vi "SP_OEE_2_test.vi"() -> ()   [LabVIEW 2017] (continued)
                      tunnel: [w12795] -> w12526
                      tunnel: [w12793] -> w12525
                      tunnel: [w12789] -> w12524
                      tunnel: [w12787] -> w12523
                      tunnel: w12538 -> [w12788]
                      tunnel: w12537 -> [w12784]
                      tunnel: [w12783] -> w12522
                      tunnel: w12536 -> [w12783]
                      tunnel: w12535 -> [w12844]
                      tunnel: w12534 -> [w12837]
                      tunnel: w12533 -> [w12828]
                      tunnel: w12532 -> [w12836]
                      tunnel: w12531 -> [w12826]
                      tunnel: w12530 -> [w12835]
                      tunnel: w12529 -> [w12824]
                      tunnel: w12528 -> [w12834]
                      tunnel: w12527 -> [w12822]
                      tunnel: w12526 -> [w12858]
                      tunnel: w12525 -> [w12857]
                      tunnel: w12524 -> [w12833]
                      tunnel: w12523 -> [w12820]
                      tunnel: [w12858] -> w12521
                      tunnel: [w12857] -> w12520
                      tunnel: [w12851] -> w12519
                      tunnel: [w12844] -> w12518
                      tunnel: [w12843] -> w12517
                      tunnel: [w12842] -> w12516
                      tunnel: [w12841] -> w12515
                      tunnel: [w12840] -> w12514
                      tunnel: [w12839] -> w12513
                      tunnel: [w12838] -> w12512
                      tunnel: [w12837] -> w12511
                      tunnel: [w12836] -> w12510
                      tunnel: [w12835] -> w12509
                      tunnel: [w12834] -> w12508
                      tunnel: [w12833] -> w12507
                      tunnel: [w12818] -> w12506
                      tunnel: w12522 -> [w12818]
                      tunnel: [w12859] -> _
                      tunnel: [w12868] -> w12497
                      tunnel: w12521 -> [w12869]
                      tunnel: w12520 -> [w12859]
                      tunnel: w12519 -> [w12863]
                      tunnel: w12518 -> [w12870]
                      tunnel: w12517 -> [_]
                      tunnel: w12516 -> [w12862]
                      tunnel: w12515 -> [_]
                      tunnel: w12514 -> [_]
                      tunnel: w12513 -> [_]
                      tunnel: w12512 -> [w12864]
                      tunnel: w12511 -> [_]
                      tunnel: w12510 -> [w12861]
                      tunnel: w12509 -> [_]
                      tunnel: w12508 -> [_]
                      tunnel: w12507 -> [_]
                      tunnel: w12506 -> [w12867]
                      tunnel: [w12859] -> w12496
                      frame #0 {
                        w12610 = "%Y-%m-%d" ("time format string (%c)")
                        n2295 = Decimal String To Number(string=w12596) -> (number=w12597:i32)  [unwired: 2 in, 1 out]
                        n2296 = property on="Table" class="Tbl (strict)"("Visible"=TRUE) -> ()  [unwired: 2 in, 2 out]
                        n2297 = Format Date/Time String(time format string (%c)=w12610, seconds (now)=w12602) -> (date/time string=w12611:string)  [unwired: 1 in]
                        n2298 = Format Date/Time String(time format string (%c)=w12610, seconds (now)=w12601) -> (date/time string=w12609:string)  [unwired: 1 in]
                        n2299 = Format Into String(format string="Where BREAKDOWN_DATE between '%s' and '%s' and  SHIFT_ID = '%d'  ", w12611, w12609, w12597) -> (resulting string=w12608:string)  [unwired: 2 in, 1 out]
                        n2300 = call <vilib>:"DB Tools Select Data.vi"("condition"=w12608, "error in (no error)"=w12617, "columns"=string[] ["BREAKDOWN_DATE"], "table"="STATION_1_LOG_HISTORY", "connection reference"=w12619) -> ("error out"=w12604:errorcluster, "data"=w12607:variant[][], "connection reference out"=w12618:T2)  [unwired: 1 in]
                        n2301 = property on="Table 2" class="Tbl (strict)"("Visible"=FALSE) -> ()  [unwired: 2 in, 2 out]
                        n2302 = xnode "Database Variant To Data"("database variant"=w12607, "error in (no error)"=w12604, "type"=string[][] [] ("Elements Found")) -> ("data"=w12605:string[][], "error out"=w12603:errorcluster)
                        n2303 = Index Array(array=w12605, index (col)=0 ("disabled index (col)")) -> (element=w12613:string[])  [unwired: 1 in]
                        n2304 = call "Search_1d_array_element.vi"("Count in"=string[] [] ("Elements Found"), "BD Date"=w12613, "Elements Found in"=string[] [] ("Elements Found")) -> ("Elements Found out"=w12600:string[])  [unwired: 4 in, 2 out]
                        n2305 = Build Array(w12600) -> (w12623:string[][])
                        n2306 = Transpose 2D Array(2D array=w12623) -> (transposed array=w12622:string[][])
                      }
                      frame #1 {
                        n2307 = disable-structure shown="Enabled" {
                          disable-tunnel: w12685 -> [w12696 w12698]
                          disable-tunnel: [w12695 w12698] -> w12684
                          disable-tunnel: w12683 -> [w12694 w12699]
                          disable-tunnel: [w12693 w12699] -> w12682
                          disable-tunnel: w12680 -> [w12691 _]
                          disable-tunnel: w12679 -> [w12690 _]
                          disable-tunnel: [w12689 _] -> w12678
                          disable-tunnel: [w12688 _] -> w12675
                          disable-tunnel: w12673 -> [w12687 _]
                          disable-tunnel: w12670 -> [w12686 w12697]
                          disable-tunnel: [_ w12697] -> w12669
                          frame Disabled {
                            n2308 = call "Stack_holderwise_total_bd_count_&_duration_2.vi"("Refnum in"=w12696, "BREAKDOWN_STK_HOLD_ID"=1, "condition"=w12687, "Form Date"=w12691, "To Date"=w12690, "error in (no error)"=w12694, "Shift"=w12686) -> ("Refnum out"=w12695:T2, "Count out"=w12689:string[], "appended array"=w12688:dbl[], "error out"=w12693:errorcluster)  [unwired: 5 in]
                          }
                          frame Enabled {
                          }
                        }
                        n2309 = call "NUMERIC TO STRING.vi"("appended array"=w12675) -> ("Array"=w12674:string[])  [unwired: 4 in]
                        n2310 = call "Insert_empty_element_with_zero.vi"("searched date"=w12678, "fixed date"=w12676) -> ("O/P"=w12671:string[])  [unwired: 9 in]
                        n2311 = call "Insert_empty_element_with_zero.vi"("searched date"=w12674, "fixed date"=w12676) -> ("O/P"=w12677:string[])  [unwired: 9 in]
                      }
                      frame #2 {
                        n2312 = call "Stack_holderwise_total_bd_count_&_duration_2.vi"("Refnum in"=w12713, "BREAKDOWN_STK_HOLD_ID"=2, "condition"=w12703, "Form Date"=w12711, "To Date"=w12710, "error in (no error)"=w12715, "Shift"=w12700) -> ("Refnum out"=w12712:T2, "Count out"=w12709:string[], "appended array"=w12705:dbl[], "error out"=w12714:errorcluster)  [unwired: 5 in]
                        n2313 = call "Insert_empty_element_with_zero.vi"("searched date"=w12709, "fixed date"=w12706) -> ("O/P"=w12708:string[])  [unwired: 9 in]
                        n2314 = call "NUMERIC TO STRING.vi"("appended array"=w12705) -> ("Array"=w12704:string[])  [unwired: 4 in]
                        n2315 = call "Insert_empty_element_with_zero.vi"("searched date"=w12704, "fixed date"=w12706) -> ("O/P"=w12707:string[])  [unwired: 9 in]
                      }
                      frame #3 {
                        n2316 = disable-structure shown="Enabled" {
                          disable-tunnel: w12732 -> [w12746 w12749]
                          disable-tunnel: [w12745 w12749] -> w12731
                          disable-tunnel: w12730 -> [w12744 w12748]
                          disable-tunnel: [w12743 w12748] -> w12729
                          disable-tunnel: w12728 -> [w12742 _]
                          disable-tunnel: w12727 -> [w12741 _]
                          disable-tunnel: [w12740 _] -> w12726
                          disable-tunnel: [w12739 _] -> w12722
                          disable-tunnel: w12720 -> [w12738 _]
                          frame Disabled {
                            n2317 = call "Stack_holderwise_total_bd_count_&_duration.vi"("Refnum in"=w12744, "BREAKDOWN_STK_HOLD_ID"=3, "condition"=w12738, "Form Date"=w12742, "To Date"=w12741, "error in (no error)"=w12746) -> ("Refnum out"=w12743:T2, "Count out"=w12740:string[], "appended array"=w12739:dbl[], "error out"=w12745:errorcluster)  [unwired: 6 in]
                          }
                          frame Enabled {
                          }
                        }
                        n2318 = call "Insert_empty_element_with_zero.vi"("searched date"=w12726, "fixed date"=w12723) -> ("O/P"=w12725:string[])  [unwired: 9 in]
                        n2319 = call "NUMERIC TO STRING.vi"("appended array"=w12722) -> ("Array"=w12721:string[])  [unwired: 4 in]
                        n2320 = call "Insert_empty_element_with_zero.vi"("searched date"=w12721, "fixed date"=w12723) -> ("O/P"=w12724:string[])  [unwired: 9 in]
                      }
                      frame #4 {
                        n2321 = disable-structure shown="Enabled" {
                          disable-tunnel: w12763 -> [w12779 w12782]
                          disable-tunnel: w12762 -> [w12778 w12781]
                          disable-tunnel: [w12777 w12781] -> w12761
                          disable-tunnel: [w12776 w12782] -> w12760
                          disable-tunnel: w12759 -> [w12775 _]
                          disable-tunnel: w12758 -> [w12774 _]
                          disable-tunnel: [w12773 _] -> w12757
                          disable-tunnel: [w12772 _] -> w12753
                          disable-tunnel: w12751 -> [w12771 _]
                          frame Disabled {
                            n2322 = call "Stack_holderwise_total_bd_count_&_duration.vi"("Refnum in"=w12778, "BREAKDOWN_STK_HOLD_ID"=4, "condition"=w12771, "Form Date"=w12775, "To Date"=w12774, "error in (no error)"=w12779) -> ("Refnum out"=w12777:T2, "Count out"=w12773:string[], "appended array"=w12772:dbl[], "error out"=w12776:errorcluster)  [unwired: 6 in]
                          }
                          frame Enabled {
                          }
                        }
                        n2323 = call "Insert_empty_element_with_zero.vi"("searched date"=w12757, "fixed date"=w12754) -> ("O/P"=w12756:string[])  [unwired: 9 in]
                        n2324 = call "NUMERIC TO STRING.vi"("appended array"=w12753) -> ("Array"=w12752:string[])  [unwired: 4 in]
                        n2325 = call "Insert_empty_element_with_zero.vi"("searched date"=w12752, "fixed date"=w12754) -> ("O/P"=w12755:string[])  [unwired: 9 in]
                      }
                      frame #5 {
                        n2326 = disable-structure shown="Enabled" {
                          disable-tunnel: w12796 -> [w12814 w12817]
                          disable-tunnel: [w12813 w12817] -> w12795
                          disable-tunnel: w12794 -> [w12812 w12816]
                          disable-tunnel: [w12811 w12816] -> w12793
                          disable-tunnel: w12792 -> [w12810 _]
                          disable-tunnel: w12791 -> [w12809 _]
                          disable-tunnel: [w12808 _] -> w12790
                          disable-tunnel: [w12807 _] -> w12786
                          disable-tunnel: w12784 -> [w12806 _]
                          frame Disabled {
                            n2327 = call "Stack_holderwise_total_bd_count_&_duration.vi"("Refnum in"=w12812, "BREAKDOWN_STK_HOLD_ID"=5, "condition"=w12806, "Form Date"=w12809, "To Date"=w12810, "error in (no error)"=w12814) -> ("Refnum out"=w12811:T2, "Count out"=w12808:string[], "appended array"=w12807:dbl[], "error out"=w12813:errorcluster)  [unwired: 6 in]
                          }
                          frame Enabled {
                          }
                        }
                        n2328 = call "NUMERIC TO STRING.vi"("appended array"=w12786) -> ("Array"=w12785:string[])  [unwired: 4 in]
                        n2329 = call "Insert_empty_element_with_zero.vi"("searched date"=w12790, "fixed date"=w12788) -> ("O/P"=w12789:string[])  [unwired: 9 in]
                        n2330 = call "Insert_empty_element_with_zero.vi"("searched date"=w12785, "fixed date"=w12788) -> ("O/P"=w12787:string[])  [unwired: 9 in]
                      }
                      frame #6 {
                        n2331 = call "String to numeric.vi"("Array"=w12828) -> ("Array 2"=w12827:dbl[])  [unwired: 4 in]
                        n2332 = call "String to numeric.vi"("Array"=w12826) -> ("Array 2"=w12825:dbl[])  [unwired: 4 in]
                        n2333 = call "String to numeric.vi"("Array"=w12824) -> ("Array 2"=w12823:dbl[])  [unwired: 4 in]
                        n2334 = call "String to numeric.vi"("Array"=w12822) -> ("Array 2"=w12821:dbl[])  [unwired: 4 in]
                        n2335 = call "String to numeric.vi"("Array"=w12820) -> ("Array 2"=w12819:dbl[])  [unwired: 4 in]
                        n2336 = Decimal String To Number(string=w12833) -> (number=w12852:i32[])  [unwired: 2 in, 1 out]
                        n2337 = Decimal String To Number(string=w12834) -> (number=w12853:i32[])  [unwired: 2 in, 1 out]
                        n2338 = Decimal String To Number(string=w12835) -> (number=w12854:i32[])  [unwired: 2 in, 1 out]
                        n2339 = Decimal String To Number(string=w12836) -> (number=w12855:i32[])  [unwired: 2 in, 1 out]
                        n2340 = Decimal String To Number(string=w12837) -> (number=w12850:i32[])  [unwired: 2 in, 1 out]
                        n2341 = Compound Arithmetic op=ADD(w12827, w12825, w12823, w12821, w12819) -> (w12830:dbl[])
                        n2342 = Build Array(w12828) -> (w12849:string[][])
                        n2343 = Build Array(w12826) -> (w12848:string[][])
                        n2344 = Build Array(w12824) -> (w12847:string[][])
                        n2345 = Build Array(w12822) -> (w12846:string[][])
                        n2346 = Build Array(w12820) -> (w12845:string[][])
                        n2347 = Number To Fractional String(number=w12830, precision (6)=i16 2) -> (F-format string=w12829:string[])  [unwired: 2 in]
                        n2348 = Compound Arithmetic op=ADD(w12852, w12853, w12854, w12855, w12850) -> (w12856:i32[])
                        n2349 = Transpose 2D Array(2D array=w12849) -> (transposed array=w12843:string[][])
                        n2350 = Transpose 2D Array(2D array=w12848) -> (transposed array=w12842:string[][])
                        n2351 = Transpose 2D Array(2D array=w12847) -> (transposed array=w12841:string[][])
                        n2352 = Transpose 2D Array(2D array=w12846) -> (transposed array=w12840:string[][])
                        n2353 = Transpose 2D Array(2D array=w12845) -> (transposed array=w12839:string[][])
                        n2354 = Number To Decimal String(number=w12856) -> (decimal integer string=w12851:string[])  [unwired: 1 in]
                        n2355 = Build Array(w12829) -> (w12832:string[][])
                        n2356 = Transpose 2D Array(2D array=w12832) -> (transposed array=w12838:string[][])
                      }
                      frame #7 {
                        w12860 = string[] [""]
                        n2357 = Insert Into Array(array=w12870, index (col)=1 ("disabled index (col)"), new element #1=w12860, new element #2=w12860, new element #3=w12861, new element #4=w12862, new element #5=w12860, new element #6=w12860, new element #7=w12860, new element #8=w12860, new element #9=w12860, new element #10=w12860, new element #11=w12863, new element #12=w12864) -> (w12866:string[][])  [unwired: 1 in]
                        n2358 = call "flot graph for month n year.vi"("BD Date"=w12867, "error in (no error)"=w12869, "Count total"=w12863) -> ("error out"=w12868:errorcluster, "Run-Time Status"=w12865:cluster{"Array 2":timestamp[], dbl[]})  [unwired: 7 in]
                        n2359 = local write "Run-Time Status"(w12865) -> ()
                        n2360 = local write "Table"(w12866) -> ()
                      }
                    }
                  }
                  frame "2" {
                    n2361 = flat-sequence {
                      tunnel: w12879 -> [w12993]
                      tunnel: w12878 -> [w12991]
                      tunnel: [w12977] -> w12969
                      tunnel: [w12992] -> w12968
                      tunnel: w12877 -> [_]
                      tunnel: [w12996] -> w12967
                      tunnel: [w12976] -> w12966
                      tunnel: [w12975] -> w12965
                      tunnel: [w12974] -> w12964
                      tunnel: w12876 -> [w12976]
                      tunnel: w12875 -> [w12975]
                      tunnel: ["Where BREAKDOWN_DATE between '%s'and '%s' and BREAKDOWN_STK_HOLD_ID ='%d' and  SHIFT_ID = '%d' "] -> w12963
                      tunnel: [w12974] -> w12962
                      tunnel: w12874 -> [w12970]
                      tunnel: [w12970] -> w12873
                      tunnel: w12969 -> [w13057]
                      tunnel: w12968 -> [w13059]
                      tunnel: w12967 -> [w13055]
                      tunnel: w12966 -> [w13054]
                      tunnel: w12965 -> [w13053]
                      tunnel: [w13056] -> w12961
                      tunnel: [w13058] -> w12960
                      tunnel: [w13055] -> w12959
                      tunnel: [w13045] -> w12958
                      tunnel: [w13051] -> w12957
                      tunnel: [w13054] -> w12956
                      tunnel: [w13053] -> w12955
                      tunnel: w12964 -> [w13050]
                      tunnel: [w13050] -> w12954
                      tunnel: w12963 -> [w13047]
                      tunnel: [w13047] -> w12953
                      tunnel: [w13046] -> w12952
                      tunnel: w12962 -> [w13046]
                      tunnel: w12873 -> [w13044]
                      tunnel: [w13043] -> w12872
                      tunnel: w12961 -> [w13089]
                      tunnel: w12960 -> [w13087]
                      tunnel: w12959 -> [w13092]
                      tunnel: w12958 -> [w13091]
                      tunnel: w12957 -> [w13090]
                      tunnel: w12956 -> [w13085]
                      tunnel: w12955 -> [w13084]
                      tunnel: [w13092] -> w12951
                      tunnel: [w13091] -> w12950
                      tunnel: [w13090] -> w12949
                      tunnel: [w13088] -> w12948
                      tunnel: [w13082] -> w12947
                      tunnel: [w13081] -> w12946
                      tunnel: [w13086] -> w12945
                      tunnel: [w13085] -> w12944
                      tunnel: [w13084] -> w12943
                      tunnel: w12954 -> [w13080]
                      tunnel: [w13080] -> w12942
                      tunnel: w12953 -> [w13077]
                      tunnel: [w13077] -> w12941
                      tunnel: [w13076] -> w12940
                      tunnel: w12952 -> [w13076]
                      tunnel: w12872 -> [w13074]
                      tunnel: w12951 -> [w13111]
                      tunnel: w12950 -> [w13110]
                      tunnel: w12949 -> [w13109]
                      tunnel: w12948 -> [w13106]
                      tunnel: w12947 -> [w13108]
                      tunnel: w12946 -> [w13107]
                      tunnel: w12945 -> [w13104]
                      tunnel: w12944 -> [w13102]
                      tunnel: w12943 -> [w13101]
                      tunnel: [w13111] -> w12939
                      tunnel: [w13110] -> w12938
                      tunnel: [w13109] -> w12937
                      tunnel: [w13108] -> w12936
                      tunnel: [w13107] -> w12935
                      tunnel: [w13105] -> w12934
                      tunnel: [w13099] -> w12933
                      tunnel: [w13098] -> w12932
                      tunnel: [w13103] -> w12931
                      tunnel: [w13102] -> w12930
                      tunnel: [w13101] -> w12929
                      tunnel: w12942 -> [w13097]
                      tunnel: [w13097] -> w12928
                      tunnel: w12941 -> [w13094]
                      tunnel: [w13094] -> w12927
                      tunnel: [w13093] -> w12926
                      tunnel: w12940 -> [w13093]
                      tunnel: w12939 -> [w13144]
                      tunnel: w12938 -> [w13143]
                      tunnel: w12937 -> [w13142]
                      tunnel: w12936 -> [w13141]
                      tunnel: w12935 -> [w13140]
                      tunnel: w12934 -> [w13137]
                      tunnel: w12933 -> [w13139]
                      tunnel: w12932 -> [w13138]
                      tunnel: w12931 -> [w13136]
                      tunnel: w12930 -> [w13133]
                      tunnel: w12929 -> [w13132]
                      tunnel: [w13144] -> w12925
                      tunnel: [w13143] -> w12924
                      tunnel: [w13142] -> w12923
                      tunnel: [w13141] -> w12922
                      tunnel: [w13140] -> w12921
                      tunnel: [w13139] -> w12920
                      tunnel: [w13138] -> w12919
                      tunnel: [w13135] -> w12918
                      tunnel: [w13134] -> w12917
                      tunnel: [w13130] -> w12916
                      tunnel: [w13129] -> w12915
                      tunnel: [w13133] -> w12914
                      tunnel: [w13132] -> w12913
                      tunnel: w12928 -> [w13128]
                      tunnel: [w13128] -> w12912
                      tunnel: w12927 -> [w13125]
                      tunnel: [w13125] -> w12911
                      tunnel: [w13124] -> w12910
                      tunnel: w12926 -> [w13124]
                      tunnel: w12925 -> [w13179]
                      tunnel: w12924 -> [w13178]
                      tunnel: w12923 -> [w13177]
                      tunnel: w12922 -> [w13176]
                      tunnel: w12921 -> [w13175]
                      tunnel: w12920 -> [w13174]
                      tunnel: w12919 -> [w13173]
                      tunnel: w12918 -> [w13168]
                      tunnel: w12917 -> [w13170]
                      tunnel: w12916 -> [w13172]
                      tunnel: w12915 -> [w13171]
                      tunnel: w12914 -> [w13165]
                      tunnel: w12913 -> [w13166]
                      tunnel: [w13179] -> w12909
                      tunnel: [w13178] -> w12908
                      tunnel: [w13177] -> w12907
                      tunnel: [w13176] -> w12906
                      tunnel: [w13175] -> w12905
                      tunnel: [w13174] -> w12904
                      tunnel: [w13173] -> w12903
                      tunnel: [w13172] -> w12902
                      tunnel: [w13171] -> w12901
                      tunnel: [w13169] -> w12900
                      tunnel: [w13167] -> w12899
                      tunnel: [w13163] -> w12898
                      tunnel: [w13161] -> w12897
                      tunnel: w12912 -> [w13162]
                      tunnel: w12911 -> [w13158]
                      tunnel: [w13157] -> w12896
                      tunnel: w12910 -> [w13157]
                      tunnel: w12909 -> [w13218]
                      tunnel: w12908 -> [w13211]
                      tunnel: w12907 -> [w13202]
                      tunnel: w12906 -> [w13210]
                      tunnel: w12905 -> [w13200]
                      tunnel: w12904 -> [w13209]
                      tunnel: w12903 -> [w13198]
                      tunnel: w12902 -> [w13208]
                      tunnel: w12901 -> [w13196]
                      tunnel: w12900 -> [w13232]
                      tunnel: w12899 -> [w13231]
                      tunnel: w12898 -> [w13207]
                      tunnel: w12897 -> [w13194]
                      tunnel: [w13232] -> w12895
                      tunnel: [w13231] -> w12894
                      tunnel: [w13225] -> w12893
                      tunnel: [w13218] -> w12892
                      tunnel: [w13217] -> w12891
                      tunnel: [w13216] -> w12890
                      tunnel: [w13215] -> w12889
                      tunnel: [w13214] -> w12888
                      tunnel: [w13213] -> w12887
                      tunnel: [w13212] -> w12886
                      tunnel: [w13211] -> w12885
                      tunnel: [w13210] -> w12884
                      tunnel: [w13209] -> w12883
                      tunnel: [w13208] -> w12882
                      tunnel: [w13207] -> w12881
                      tunnel: [w13192] -> w12880
                      tunnel: w12896 -> [w13192]
                      tunnel: [w13245] -> _
                      tunnel: [w13241] -> _
                      tunnel: w12895 -> [w13242]
                      tunnel: w12894 -> [w13245]
                      tunnel: w12893 -> [w13236]
                      tunnel: w12892 -> [w13243]
                      tunnel: w12891 -> [_]
                      tunnel: w12890 -> [w13235]
                      tunnel: w12889 -> [_]
                      tunnel: w12888 -> [_]
                      tunnel: w12887 -> [_]
                      tunnel: w12886 -> [w13237]
                      tunnel: w12885 -> [_]
                      tunnel: w12884 -> [w13234]
                      tunnel: w12883 -> [_]
                      tunnel: w12882 -> [_]
                      tunnel: w12881 -> [_]
                      tunnel: w12880 -> [w13240]
                      frame #0 {
                        w12984 = "%Y-%m-%d" ("time format string (%c)")
                        n2362 = Decimal String To Number(string=w12970) -> (number=w12971:i32)  [unwired: 2 in, 1 out]
                        n2363 = property on="Table" class="Tbl (strict)"("Visible"=TRUE) -> ()  [unwired: 2 in, 2 out]
                        n2364 = Format Date/Time String(time format string (%c)=w12984, seconds (now)=w12976) -> (date/time string=w12985:string)  [unwired: 1 in]
                        n2365 = Format Date/Time String(time format string (%c)=w12984, seconds (now)=w12975) -> (date/time string=w12983:string)  [unwired: 1 in]
                        n2366 = Format Into String(format string="Where BREAKDOWN_DATE between '%s' and '%s' and  SHIFT_ID = '%d'  ", w12985, w12983, w12971) -> (resulting string=w12982:string)  [unwired: 2 in, 1 out]
                        n2367 = call <vilib>:"DB Tools Select Data.vi"("condition"=w12982, "error in (no error)"=w12991, "columns"=string[] ["BREAKDOWN_DATE"], "table"="STATION_1_LOG_HISTORY", "connection reference"=w12993) -> ("error out"=w12978:errorcluster, "data"=w12981:variant[][], "connection reference out"=w12992:T2)  [unwired: 1 in]
                        n2368 = property on="Table 2" class="Tbl (strict)"("Visible"=FALSE) -> ()  [unwired: 2 in, 2 out]
                        n2369 = xnode "Database Variant To Data"("database variant"=w12981, "error in (no error)"=w12978, "type"=string[][] [] ("Elements Found")) -> ("data"=w12979:string[][], "error out"=w12977:errorcluster)
                        n2370 = Index Array(array=w12979, index (col)=0 ("disabled index (col)")) -> (element=w12987:string[])  [unwired: 1 in]
                        n2371 = call "Search_1d_array_element.vi"("Count in"=string[] [] ("Elements Found"), "BD Date"=w12987, "Elements Found in"=string[] [] ("Elements Found")) -> ("Elements Found out"=w12974:string[])  [unwired: 4 in, 2 out]
                        n2372 = Build Array(w12974) -> (w12997:string[][])
                        n2373 = Transpose 2D Array(2D array=w12997) -> (transposed array=w12996:string[][])
                      }
                      frame #1 {
                        n2374 = disable-structure shown="Enabled" {
                          disable-tunnel: w13059 -> [w13070 w13072]
                          disable-tunnel: [w13069 w13072] -> w13058
                          disable-tunnel: w13057 -> [w13068 w13073]
                          disable-tunnel: [w13067 w13073] -> w13056
                          disable-tunnel: w13054 -> [w13065 _]
                          disable-tunnel: w13053 -> [w13064 _]
                          disable-tunnel: [w13063 _] -> w13052
                          disable-tunnel: [w13062 _] -> w13049
                          disable-tunnel: w13047 -> [w13061 _]
                          disable-tunnel: w13044 -> [w13060 w13071]
                          disable-tunnel: [_ w13071] -> w13043
                          frame Disabled {
                            n2375 = call "Stack_holderwise_total_bd_count_&_duration_2.vi"("Refnum in"=w13070, "BREAKDOWN_STK_HOLD_ID"=1, "condition"=w13061, "Form Date"=w13065, "To Date"=w13064, "error in (no error)"=w13068, "Shift"=w13060) -> ("Refnum out"=w13069:T2, "Count out"=w13063:string[], "appended array"=w13062:dbl[], "error out"=w13067:errorcluster)  [unwired: 5 in]
                          }
                          frame Enabled {
                          }
                        }
                        n2376 = call "NUMERIC TO STRING.vi"("appended array"=w13049) -> ("Array"=w13048:string[])  [unwired: 4 in]
                        n2377 = call "Insert_empty_element_with_zero.vi"("searched date"=w13052, "fixed date"=w13050) -> ("O/P"=w13045:string[])  [unwired: 9 in]
                        n2378 = call "Insert_empty_element_with_zero.vi"("searched date"=w13048, "fixed date"=w13050) -> ("O/P"=w13051:string[])  [unwired: 9 in]
                      }
                      frame #2 {
                        n2379 = call "Stack_holderwise_total_bd_count_&_duration_2.vi"("Refnum in"=w13087, "BREAKDOWN_STK_HOLD_ID"=2, "condition"=w13077, "Form Date"=w13085, "To Date"=w13084, "error in (no error)"=w13089, "Shift"=w13074) -> ("Refnum out"=w13086:T2, "Count out"=w13083:string[], "appended array"=w13079:dbl[], "error out"=w13088:errorcluster)  [unwired: 5 in]
                        n2380 = call "Insert_empty_element_with_zero.vi"("searched date"=w13083, "fixed date"=w13080) -> ("O/P"=w13082:string[])  [unwired: 9 in]
                        n2381 = call "NUMERIC TO STRING.vi"("appended array"=w13079) -> ("Array"=w13078:string[])  [unwired: 4 in]
                        n2382 = call "Insert_empty_element_with_zero.vi"("searched date"=w13078, "fixed date"=w13080) -> ("O/P"=w13081:string[])  [unwired: 9 in]
                      }
                      frame #3 {
                        n2383 = disable-structure shown="Enabled" {
                          disable-tunnel: w13106 -> [w13120 w13123]
                          disable-tunnel: [w13119 w13123] -> w13105
                          disable-tunnel: w13104 -> [w13118 w13122]
                          disable-tunnel: [w13117 w13122] -> w13103
                          disable-tunnel: w13102 -> [w13116 _]
                          disable-tunnel: w13101 -> [w13115 _]
                          disable-tunnel: [w13114 _] -> w13100
                          disable-tunnel: [w13113 _] -> w13096
                          disable-tunnel: w13094 -> [w13112 _]
                          frame Disabled {
                            n2384 = call "Stack_holderwise_total_bd_count_&_duration.vi"("Refnum in"=w13118, "BREAKDOWN_STK_HOLD_ID"=3, "condition"=w13112, "Form Date"=w13116, "To Date"=w13115, "error in (no error)"=w13120) -> ("Refnum out"=w13117:T2, "Count out"=w13114:string[], "appended array"=w13113:dbl[], "error out"=w13119:errorcluster)  [unwired: 6 in]
                          }
                          frame Enabled {
                          }
                        }
                        n2385 = call "Insert_empty_element_with_zero.vi"("searched date"=w13100, "fixed date"=w13097) -> ("O/P"=w13099:string[])  [unwired: 9 in]
                        n2386 = call "NUMERIC TO STRING.vi"("appended array"=w13096) -> ("Array"=w13095:string[])  [unwired: 4 in]
                        n2387 = call "Insert_empty_element_with_zero.vi"("searched date"=w13095, "fixed date"=w13097) -> ("O/P"=w13098:string[])  [unwired: 9 in]
                      }
                      frame #4 {
                        n2388 = disable-structure shown="Enabled" {
                          disable-tunnel: w13137 -> [w13153 w13156]
                          disable-tunnel: w13136 -> [w13152 w13155]
                          disable-tunnel: [w13151 w13155] -> w13135
                          disable-tunnel: [w13150 w13156] -> w13134
                          disable-tunnel: w13133 -> [w13149 _]
                          disable-tunnel: w13132 -> [w13148 _]
                          disable-tunnel: [w13147 _] -> w13131
                          disable-tunnel: [w13146 _] -> w13127
                          disable-tunnel: w13125 -> [w13145 _]
                          frame Disabled {
                            n2389 = call "Stack_holderwise_total_bd_count_&_duration.vi"("Refnum in"=w13152, "BREAKDOWN_STK_HOLD_ID"=4, "condition"=w13145, "Form Date"=w13149, "To Date"=w13148, "error in (no error)"=w13153) -> ("Refnum out"=w13151:T2, "Count out"=w13147:string[], "appended array"=w13146:dbl[], "error out"=w13150:errorcluster)  [unwired: 6 in]
                          }
                          frame Enabled {
                          }
                        }
                        n2390 = call "Insert_empty_element_with_zero.vi"("searched date"=w13131, "fixed date"=w13128) -> ("O/P"=w13130:string[])  [unwired: 9 in]
                        n2391 = call "NUMERIC TO STRING.vi"("appended array"=w13127) -> ("Array"=w13126:string[])  [unwired: 4 in]
                        n2392 = call "Insert_empty_element_with_zero.vi"("searched date"=w13126, "fixed date"=w13128) -> ("O/P"=w13129:string[])  [unwired: 9 in]
                      }
                      frame #5 {
                        n2393 = disable-structure shown="Enabled" {
                          disable-tunnel: w13170 -> [w13188 w13191]
                          disable-tunnel: [w13187 w13191] -> w13169
                          disable-tunnel: w13168 -> [w13186 w13190]
                          disable-tunnel: [w13185 w13190] -> w13167
                          disable-tunnel: w13166 -> [w13184 _]
                          disable-tunnel: w13165 -> [w13183 _]
                          disable-tunnel: [w13182 _] -> w13164
                          disable-tunnel: [w13181 _] -> w13160
                          disable-tunnel: w13158 -> [w13180 _]
                          frame Disabled {
                            n2394 = call "Stack_holderwise_total_bd_count_&_duration.vi"("Refnum in"=w13186, "BREAKDOWN_STK_HOLD_ID"=5, "condition"=w13180, "Form Date"=w13183, "To Date"=w13184, "error in (no error)"=w13188) -> ("Refnum out"=w13185:T2, "Count out"=w13182:string[], "appended array"=w13181:dbl[], "error out"=w13187:errorcluster)  [unwired: 6 in]
                          }
                          frame Enabled {
                          }
                        }
                        n2395 = call "NUMERIC TO STRING.vi"("appended array"=w13160) -> ("Array"=w13159:string[])  [unwired: 4 in]
                        n2396 = call "Insert_empty_element_with_zero.vi"("searched date"=w13164, "fixed date"=w13162) -> ("O/P"=w13163:string[])  [unwired: 9 in]
                        n2397 = call "Insert_empty_element_with_zero.vi"("searched date"=w13159, "fixed date"=w13162) -> ("O/P"=w13161:string[])  [unwired: 9 in]
                      }
                      frame #6 {
                        n2398 = call "String to numeric.vi"("Array"=w13202) -> ("Array 2"=w13201:dbl[])  [unwired: 4 in]
                        n2399 = call "String to numeric.vi"("Array"=w13200) -> ("Array 2"=w13199:dbl[])  [unwired: 4 in]
                        n2400 = call "String to numeric.vi"("Array"=w13198) -> ("Array 2"=w13197:dbl[])  [unwired: 4 in]
                        n2401 = call "String to numeric.vi"("Array"=w13196) -> ("Array 2"=w13195:dbl[])  [unwired: 4 in]
                        n2402 = call "String to numeric.vi"("Array"=w13194) -> ("Array 2"=w13193:dbl[])  [unwired: 4 in]
                        n2403 = Decimal String To Number(string=w13207) -> (number=w13226:i32[])  [unwired: 2 in, 1 out]
                        n2404 = Decimal String To Number(string=w13208) -> (number=w13227:i32[])  [unwired: 2 in, 1 out]
                        n2405 = Decimal String To Number(string=w13209) -> (number=w13228:i32[])  [unwired: 2 in, 1 out]
                        n2406 = Decimal String To Number(string=w13210) -> (number=w13229:i32[])  [unwired: 2 in, 1 out]
                        n2407 = Decimal String To Number(string=w13211) -> (number=w13224:i32[])  [unwired: 2 in, 1 out]
                        n2408 = Compound Arithmetic op=ADD(w13201, w13199, w13197, w13195, w13193) -> (w13204:dbl[])
                        n2409 = Build Array(w13202) -> (w13223:string[][])
                        n2410 = Build Array(w13200) -> (w13222:string[][])
                        n2411 = Build Array(w13198) -> (w13221:string[][])
                        n2412 = Build Array(w13196) -> (w13220:string[][])
                        n2413 = Build Array(w13194) -> (w13219:string[][])
                        n2414 = Number To Fractional String(number=w13204, precision (6)=i16 2) -> (F-format string=w13203:string[])  [unwired: 2 in]
                        n2415 = Compound Arithmetic op=ADD(w13226, w13227, w13228, w13229, w13224) -> (w13230:i32[])
                        n2416 = Transpose 2D Array(2D array=w13223) -> (transposed array=w13217:string[][])
                        n2417 = Transpose 2D Array(2D array=w13222) -> (transposed array=w13216:string[][])
                        n2418 = Transpose 2D Array(2D array=w13221) -> (transposed array=w13215:string[][])
                        n2419 = Transpose 2D Array(2D array=w13220) -> (transposed array=w13214:string[][])
                        n2420 = Transpose 2D Array(2D array=w13219) -> (transposed array=w13213:string[][])
                        n2421 = Number To Decimal String(number=w13230) -> (decimal integer string=w13225:string[])  [unwired: 1 in]
                        n2422 = Build Array(w13203) -> (w13206:string[][])
                        n2423 = Transpose 2D Array(2D array=w13206) -> (transposed array=w13212:string[][])
                      }
                      frame #7 {
                        w13233 = string[] [""]
                        n2424 = Insert Into Array(array=w13243, index (col)=1 ("disabled index (col)"), new element #1=w13233, new element #2=w13233, new element #3=w13234, new element #4=w13235, new element #5=w13233, new element #6=w13233, new element #7=w13233, new element #8=w13233, new element #9=w13233, new element #10=w13233, new element #11=w13236, new element #12=w13237) -> (w13239:string[][])  [unwired: 1 in]
                        n2425 = call "flot graph for month n year.vi"("BD Date"=w13240, "error in (no error)"=w13242, "Count total"=w13236) -> ("error out"=w13241:errorcluster, "Run-Time Status"=w13238:cluster{"Array 2":timestamp[], dbl[]})  [unwired: 7 in]
                        n2426 = local write "Run-Time Status"(w13238) -> ()
                        n2427 = local write "Table"(w13239) -> ()
                      }
                    }
                  }
                  frame "3" {
                    n2428 = flat-sequence {
                      tunnel: w13253 -> [w13367]
                      tunnel: w13252 -> [w13365]
                      tunnel: [w13351] -> w13343
                      tunnel: [w13366] -> w13342
                      tunnel: w13251 -> [_]
                      tunnel: [w13370] -> w13341
                      tunnel: [w13350] -> w13340
                      tunnel: [w13349] -> w13339
                      tunnel: [w13348] -> w13338
                      tunnel: w13250 -> [w13350]
                      tunnel: w13249 -> [w13349]
                      tunnel: ["Where BREAKDOWN_DATE between '%s'and '%s' and BREAKDOWN_STK_HOLD_ID ='%d' and  SHIFT_ID = '%d' "] -> w13337
                      tunnel: [w13348] -> w13336
                      tunnel: w13248 -> [w13344]
                      tunnel: [w13344] -> w13247
                      tunnel: w13343 -> [w13431]
                      tunnel: w13342 -> [w13433]
                      tunnel: w13341 -> [w13429]
                      tunnel: w13340 -> [w13428]
                      tunnel: w13339 -> [w13427]
                      tunnel: [w13430] -> w13335
                      tunnel: [w13432] -> w13334
                      tunnel: [w13429] -> w13333
                      tunnel: [w13419] -> w13332
                      tunnel: [w13425] -> w13331
                      tunnel: [w13428] -> w13330
                      tunnel: [w13427] -> w13329
                      tunnel: w13338 -> [w13424]
                      tunnel: [w13424] -> w13328
                      tunnel: w13337 -> [w13421]
                      tunnel: [w13421] -> w13327
                      tunnel: [w13420] -> w13326
                      tunnel: w13336 -> [w13420]
                      tunnel: w13247 -> [w13418]
                      tunnel: [w13417] -> w13246
                      tunnel: w13335 -> [w13463]
                      tunnel: w13334 -> [w13461]
                      tunnel: w13333 -> [w13466]
                      tunnel: w13332 -> [w13465]
                      tunnel: w13331 -> [w13464]
                      tunnel: w13330 -> [w13459]
                      tunnel: w13329 -> [w13458]
                      tunnel: [w13466] -> w13325
                      tunnel: [w13465] -> w13324
                      tunnel: [w13464] -> w13323
                      tunnel: [w13462] -> w13322
                      tunnel: [w13456] -> w13321
                      tunnel: [w13455] -> w13320
                      tunnel: [w13460] -> w13319
                      tunnel: [w13459] -> w13318
                      tunnel: [w13458] -> w13317
                      tunnel: w13328 -> [w13454]
                      tunnel: [w13454] -> w13316
                      tunnel: w13327 -> [w13451]
                      tunnel: [w13451] -> w13315
                      tunnel: [w13450] -> w13314
                      tunnel: w13326 -> [w13450]
                      tunnel: w13246 -> [w13448]
                      tunnel: w13325 -> [w13485]
                      tunnel: w13324 -> [w13484]
                      tunnel: w13323 -> [w13483]
                      tunnel: w13322 -> [w13480]
                      tunnel: w13321 -> [w13482]
                      tunnel: w13320 -> [w13481]
                      tunnel: w13319 -> [w13478]
                      tunnel: w13318 -> [w13476]
                      tunnel: w13317 -> [w13475]
                      tunnel: [w13485] -> w13313
                      tunnel: [w13484] -> w13312
                      tunnel: [w13483] -> w13311
                      tunnel: [w13482] -> w13310
                      tunnel: [w13481] -> w13309
                      tunnel: [w13479] -> w13308
                      tunnel: [w13473] -> w13307
                      tunnel: [w13472] -> w13306
                      tunnel: [w13477] -> w13305
                      tunnel: [w13476] -> w13304
                      tunnel: [w13475] -> w13303
                      tunnel: w13316 -> [w13471]
                      tunnel: [w13471] -> w13302
                      tunnel: w13315 -> [w13468]
                      tunnel: [w13468] -> w13301
                      tunnel: [w13467] -> w13300
                      tunnel: w13314 -> [w13467]
                      tunnel: w13313 -> [w13518]
                      tunnel: w13312 -> [w13517]
                      tunnel: w13311 -> [w13516]
                      tunnel: w13310 -> [w13515]
                      tunnel: w13309 -> [w13514]
                      tunnel: w13308 -> [w13511]
                      tunnel: w13307 -> [w13513]
                      tunnel: w13306 -> [w13512]
                      tunnel: w13305 -> [w13510]
                      tunnel: w13304 -> [w13507]
                      tunnel: w13303 -> [w13506]
                      tunnel: [w13518] -> w13299
                      tunnel: [w13517] -> w13298
                      tunnel: [w13516] -> w13297
                      tunnel: [w13515] -> w13296
                      tunnel: [w13514] -> w13295
                      tunnel: [w13513] -> w13294
                      tunnel: [w13512] -> w13293
                      tunnel: [w13509] -> w13292
                      tunnel: [w13508] -> w13291
                      tunnel: [w13504] -> w13290
                      tunnel: [w13503] -> w13289
                      tunnel: [w13507] -> w13288
                      tunnel: [w13506] -> w13287
                      tunnel: w13302 -> [w13502]
                      tunnel: [w13502] -> w13286
                      tunnel: w13301 -> [w13499]
                      tunnel: [w13499] -> w13285
                      tunnel: [w13498] -> w13284
                      tunnel: w13300 -> [w13498]
                      tunnel: w13299 -> [w13553]
                      tunnel: w13298 -> [w13552]
                      tunnel: w13297 -> [w13551]
                      tunnel: w13296 -> [w13550]
                      tunnel: w13295 -> [w13549]
                      tunnel: w13294 -> [w13548]
                      tunnel: w13293 -> [w13547]
                      tunnel: w13292 -> [w13542]
                      tunnel: w13291 -> [w13544]
                      tunnel: w13290 -> [w13546]
                      tunnel: w13289 -> [w13545]
                      tunnel: w13288 -> [w13539]
                      tunnel: w13287 -> [w13540]
                      tunnel: [w13553] -> w13283
                      tunnel: [w13552] -> w13282
                      tunnel: [w13551] -> w13281
                      tunnel: [w13550] -> w13280
                      tunnel: [w13549] -> w13279
                      tunnel: [w13548] -> w13278
                      tunnel: [w13547] -> w13277
                      tunnel: [w13546] -> w13276
                      tunnel: [w13545] -> w13275
                      tunnel: [w13543] -> w13274
                      tunnel: [w13541] -> w13273
                      tunnel: [w13537] -> w13272
                      tunnel: [w13535] -> w13271
                      tunnel: w13286 -> [w13536]
                      tunnel: w13285 -> [w13532]
                      tunnel: [w13531] -> w13270
                      tunnel: w13284 -> [w13531]
                      tunnel: w13283 -> [w13592]
                      tunnel: w13282 -> [w13585]
                      tunnel: w13281 -> [w13576]
                      tunnel: w13280 -> [w13584]
                      tunnel: w13279 -> [w13574]
                      tunnel: w13278 -> [w13583]
                      tunnel: w13277 -> [w13572]
                      tunnel: w13276 -> [w13582]
                      tunnel: w13275 -> [w13570]
                      tunnel: w13274 -> [w13606]
                      tunnel: w13273 -> [w13605]
                      tunnel: w13272 -> [w13581]
                      tunnel: w13271 -> [w13568]
                      tunnel: [w13606] -> w13269
                      tunnel: [w13605] -> w13268
                      tunnel: [w13599] -> w13267
                      tunnel: [w13592] -> w13266
                      tunnel: [w13591] -> w13265
                      tunnel: [w13590] -> w13264
                      tunnel: [w13589] -> w13263
                      tunnel: [w13588] -> w13262
                      tunnel: [w13587] -> w13261
                      tunnel: [w13586] -> w13260
                      tunnel: [w13585] -> w13259
                      tunnel: [w13584] -> w13258
                      tunnel: [w13583] -> w13257
                      tunnel: [w13582] -> w13256
                      tunnel: [w13581] -> w13255
                      tunnel: [w13566] -> w13254
                      tunnel: w13270 -> [w13566]
                      tunnel: [w13619] -> _
                      tunnel: [w13615] -> _
                      tunnel: w13269 -> [w13616]
                      tunnel: w13268 -> [w13619]
                      tunnel: w13267 -> [w13610]
                      tunnel: w13266 -> [w13617]
                      tunnel: w13265 -> [_]
                      tunnel: w13264 -> [w13609]
                      tunnel: w13263 -> [_]
                      tunnel: w13262 -> [_]
                      tunnel: w13261 -> [_]
                      tunnel: w13260 -> [w13611]
                      tunnel: w13259 -> [_]
                      tunnel: w13258 -> [w13608]
                      tunnel: w13257 -> [_]
                      tunnel: w13256 -> [_]
                      tunnel: w13255 -> [_]
                      tunnel: w13254 -> [w13614]
                      frame #0 {
                        w13358 = "%Y-%m-%d" ("time format string (%c)")
                        n2429 = Decimal String To Number(string=w13344) -> (number=w13345:i32)  [unwired: 2 in, 1 out]
                        n2430 = property on="Table" class="Tbl (strict)"("Visible"=TRUE) -> ()  [unwired: 2 in, 2 out]
                        n2431 = Format Date/Time String(time format string (%c)=w13358, seconds (now)=w13350) -> (date/time string=w13359:string)  [unwired: 1 in]
                        n2432 = Format Date/Time String(time format string (%c)=w13358, seconds (now)=w13349) -> (date/time string=w13357:string)  [unwired: 1 in]
                        n2433 = Format Into String(format string="Where BREAKDOWN_DATE between '%s' and '%s' and  SHIFT_ID = '%d'  ", w13359, w13357, w13345) -> (resulting string=w13356:string)  [unwired: 2 in, 1 out]
                        n2434 = call <vilib>:"DB Tools Select Data.vi"("condition"=w13356, "error in (no error)"=w13365, "columns"=string[] ["BREAKDOWN_DATE"], "table"="STATION_1_LOG_HISTORY", "connection reference"=w13367) -> ("error out"=w13352:errorcluster, "data"=w13355:variant[][], "connection reference out"=w13366:T2)  [unwired: 1 in]
                        n2435 = property on="Table 2" class="Tbl (strict)"("Visible"=FALSE) -> ()  [unwired: 2 in, 2 out]
                        n2436 = xnode "Database Variant To Data"("database variant"=w13355, "error in (no error)"=w13352, "type"=string[][] [] ("Elements Found")) -> ("data"=w13353:string[][], "error out"=w13351:errorcluster)
                        n2437 = Index Array(array=w13353, index (col)=0 ("disabled index (col)")) -> (element=w13361:string[])  [unwired: 1 in]
                        n2438 = call "Search_1d_array_element.vi"("Count in"=string[] [] ("Elements Found"), "BD Date"=w13361, "Elements Found in"=string[] [] ("Elements Found")) -> ("Elements Found out"=w13348:string[])  [unwired: 4 in, 2 out]
                        n2439 = Build Array(w13348) -> (w13371:string[][])
                        n2440 = Transpose 2D Array(2D array=w13371) -> (transposed array=w13370:string[][])
                      }
                      frame #1 {
                        n2441 = disable-structure shown="Enabled" {
                          disable-tunnel: w13433 -> [w13444 w13446]
                          disable-tunnel: [w13443 w13446] -> w13432
                          disable-tunnel: w13431 -> [w13442 w13447]
                          disable-tunnel: [w13441 w13447] -> w13430
                          disable-tunnel: w13428 -> [w13439 _]
                          disable-tunnel: w13427 -> [w13438 _]
                          disable-tunnel: [w13437 _] -> w13426
                          disable-tunnel: [w13436 _] -> w13423
                          disable-tunnel: w13421 -> [w13435 _]
                          disable-tunnel: w13418 -> [w13434 w13445]
                          disable-tunnel: [_ w13445] -> w13417
                          frame Disabled {
                            n2442 = call "Stack_holderwise_total_bd_count_&_duration_2.vi"("Refnum in"=w13444, "BREAKDOWN_STK_HOLD_ID"=1, "condition"=w13435, "Form Date"=w13439, "To Date"=w13438, "error in (no error)"=w13442, "Shift"=w13434) -> ("Refnum out"=w13443:T2, "Count out"=w13437:string[], "appended array"=w13436:dbl[], "error out"=w13441:errorcluster)  [unwired: 5 in]
                          }
                          frame Enabled {
                          }
                        }
                        n2443 = call "NUMERIC TO STRING.vi"("appended array"=w13423) -> ("Array"=w13422:string[])  [unwired: 4 in]
                        n2444 = call "Insert_empty_element_with_zero.vi"("searched date"=w13426, "fixed date"=w13424) -> ("O/P"=w13419:string[])  [unwired: 9 in]
                        n2445 = call "Insert_empty_element_with_zero.vi"("searched date"=w13422, "fixed date"=w13424) -> ("O/P"=w13425:string[])  [unwired: 9 in]
                      }
                      frame #2 {
                        n2446 = call "Stack_holderwise_total_bd_count_&_duration_2.vi"("Refnum in"=w13461, "BREAKDOWN_STK_HOLD_ID"=2, "condition"=w13451, "Form Date"=w13459, "To Date"=w13458, "error in (no error)"=w13463, "Shift"=w13448) -> ("Refnum out"=w13460:T2, "Count out"=w13457:string[], "appended array"=w13453:dbl[], "error out"=w13462:errorcluster)  [unwired: 5 in]
                        n2447 = call "Insert_empty_element_with_zero.vi"("searched date"=w13457, "fixed date"=w13454) -> ("O/P"=w13456:string[])  [unwired: 9 in]
                        n2448 = call "NUMERIC TO STRING.vi"("appended array"=w13453) -> ("Array"=w13452:string[])  [unwired: 4 in]
                        n2449 = call "Insert_empty_element_with_zero.vi"("searched date"=w13452, "fixed date"=w13454) -> ("O/P"=w13455:string[])  [unwired: 9 in]
                      }
                      frame #3 {
                        n2450 = disable-structure shown="Enabled" {
                          disable-tunnel: w13480 -> [w13494 w13497]
                          disable-tunnel: [w13493 w13497] -> w13479
                          disable-tunnel: w13478 -> [w13492 w13496]
                          disable-tunnel: [w13491 w13496] -> w13477
                          disable-tunnel: w13476 -> [w13490 _]
                          disable-tunnel: w13475 -> [w13489 _]
                          disable-tunnel: [w13488 _] -> w13474
                          disable-tunnel: [w13487 _] -> w13470
                          disable-tunnel: w13468 -> [w13486 _]
                          frame Disabled {
                            n2451 = call "Stack_holderwise_total_bd_count_&_duration.vi"("Refnum in"=w13492, "BREAKDOWN_STK_HOLD_ID"=3, "condition"=w13486, "Form Date"=w13490, "To Date"=w13489, "error in (no error)"=w13494) -> ("Refnum out"=w13491:T2, "Count out"=w13488:string[], "appended array"=w13487:dbl[], "error out"=w13493:errorcluster)  [unwired: 6 in]
                          }
                          frame Enabled {
                          }
                        }
                        n2452 = call "Insert_empty_element_with_zero.vi"("searched date"=w13474, "fixed date"=w13471) -> ("O/P"=w13473:string[])  [unwired: 9 in]
                        n2453 = call "NUMERIC TO STRING.vi"("appended array"=w13470) -> ("Array"=w13469:string[])  [unwired: 4 in]
                        n2454 = call "Insert_empty_element_with_zero.vi"("searched date"=w13469, "fixed date"=w13471) -> ("O/P"=w13472:string[])  [unwired: 9 in]
                      }
                      frame #4 {
                        n2455 = disable-structure shown="Enabled" {
                          disable-tunnel: w13511 -> [w13527 w13530]
                          disable-tunnel: w13510 -> [w13526 w13529]
                          disable-tunnel: [w13525 w13529] -> w13509
                          disable-tunnel: [w13524 w13530] -> w13508
                          disable-tunnel: w13507 -> [w13523 _]
                          disable-tunnel: w13506 -> [w13522 _]
                          disable-tunnel: [w13521 _] -> w13505
                          disable-tunnel: [w13520 _] -> w13501
                          disable-tunnel: w13499 -> [w13519 _]
                          frame Disabled {
                            n2456 = call "Stack_holderwise_total_bd_count_&_duration.vi"("Refnum in"=w13526, "BREAKDOWN_STK_HOLD_ID"=4, "condition"=w13519, "Form Date"=w13523, "To Date"=w13522, "error in (no error)"=w13527) -> ("Refnum out"=w13525:T2, "Count out"=w13521:string[], "appended array"=w13520:dbl[], "error out"=w13524:errorcluster)  [unwired: 6 in]
                          }
                          frame Enabled {
                          }
                        }
                        n2457 = call "Insert_empty_element_with_zero.vi"("searched date"=w13505, "fixed date"=w13502) -> ("O/P"=w13504:string[])  [unwired: 9 in]
                        n2458 = call "NUMERIC TO STRING.vi"("appended array"=w13501) -> ("Array"=w13500:string[])  [unwired: 4 in]
                        n2459 = call "Insert_empty_element_with_zero.vi"("searched date"=w13500, "fixed date"=w13502) -> ("O/P"=w13503:string[])  [unwired: 9 in]
                      }
                      frame #5 {
                        n2460 = disable-structure shown="Enabled" {
                          disable-tunnel: w13544 -> [w13562 w13565]
                          disable-tunnel: [w13561 w13565] -> w13543
                          disable-tunnel: w13542 -> [w13560 w13564]
                          disable-tunnel: [w13559 w13564] -> w13541
                          disable-tunnel: w13540 -> [w13558 _]
                          disable-tunnel: w13539 -> [w13557 _]
                          disable-tunnel: [w13556 _] -> w13538
                          disable-tunnel: [w13555 _] -> w13534
                          disable-tunnel: w13532 -> [w13554 _]
                          frame Disabled {
                            n2461 = call "Stack_holderwise_total_bd_count_&_duration.vi"("Refnum in"=w13560, "BREAKDOWN_STK_HOLD_ID"=5, "condition"=w13554, "Form Date"=w13557, "To Date"=w13558, "error in (no error)"=w13562) -> ("Refnum out"=w13559:T2, "Count out"=w13556:string[], "appended array"=w13555:dbl[], "error out"=w13561:errorcluster)  [unwired: 6 in]
                          }
                          frame Enabled {
                          }
                        }
                        n2462 = call "NUMERIC TO STRING.vi"("appended array"=w13534) -> ("Array"=w13533:string[])  [unwired: 4 in]
                        n2463 = call "Insert_empty_element_with_zero.vi"("searched date"=w13538, "fixed date"=w13536) -> ("O/P"=w13537:string[])  [unwired: 9 in]
                        n2464 = call "Insert_empty_element_with_zero.vi"("searched date"=w13533, "fixed date"=w13536) -> ("O/P"=w13535:string[])  [unwired: 9 in]
                      }
                      frame #6 {
                        n2465 = call "String to numeric.vi"("Array"=w13576) -> ("Array 2"=w13575:dbl[])  [unwired: 4 in]
                        n2466 = call "String to numeric.vi"("Array"=w13574) -> ("Array 2"=w13573:dbl[])  [unwired: 4 in]
                        n2467 = call "String to numeric.vi"("Array"=w13572) -> ("Array 2"=w13571:dbl[])  [unwired: 4 in]
                        n2468 = call "String to numeric.vi"("Array"=w13570) -> ("Array 2"=w13569:dbl[])  [unwired: 4 in]
                        n2469 = call "String to numeric.vi"("Array"=w13568) -> ("Array 2"=w13567:dbl[])  [unwired: 4 in]
                        n2470 = Decimal String To Number(string=w13581) -> (number=w13600:i32[])  [unwired: 2 in, 1 out]
                        n2471 = Decimal String To Number(string=w13582) -> (number=w13601:i32[])  [unwired: 2 in, 1 out]
                        n2472 = Decimal String To Number(string=w13583) -> (number=w13602:i32[])  [unwired: 2 in, 1 out]
                        n2473 = Decimal String To Number(string=w13584) -> (number=w13603:i32[])  [unwired: 2 in, 1 out]
                        n2474 = Decimal String To Number(string=w13585) -> (number=w13598:i32[])  [unwired: 2 in, 1 out]
                        n2475 = Compound Arithmetic op=ADD(w13575, w13573, w13571, w13569, w13567) -> (w13578:dbl[])
                        n2476 = Build Array(w13576) -> (w13597:string[][])
                        n2477 = Build Array(w13574) -> (w13596:string[][])
                        n2478 = Build Array(w13572) -> (w13595:string[][])
                        n2479 = Build Array(w13570) -> (w13594:string[][])
                        n2480 = Build Array(w13568) -> (w13593:string[][])
                        n2481 = Number To Fractional String(number=w13578, precision (6)=i16 2) -> (F-format string=w13577:string[])  [unwired: 2 in]
                        n2482 = Compound Arithmetic op=ADD(w13600, w13601, w13602, w13603, w13598) -> (w13604:i32[])
                        n2483 = Transpose 2D Array(2D array=w13597) -> (transposed array=w13591:string[][])
                        n2484 = Transpose 2D Array(2D array=w13596) -> (transposed array=w13590:string[][])
                        n2485 = Transpose 2D Array(2D array=w13595) -> (transposed array=w13589:string[][])
                        n2486 = Transpose 2D Array(2D array=w13594) -> (transposed array=w13588:string[][])
                        n2487 = Transpose 2D Array(2D array=w13593) -> (transposed array=w13587:string[][])
                        n2488 = Number To Decimal String(number=w13604) -> (decimal integer string=w13599:string[])  [unwired: 1 in]
                        n2489 = Build Array(w13577) -> (w13580:string[][])
                        n2490 = Transpose 2D Array(2D array=w13580) -> (transposed array=w13586:string[][])
                      }
                      frame #7 {
                        w13607 = string[] [""]
                        n2491 = Insert Into Array(array=w13617, index (col)=1 ("disabled index (col)"), new element #1=w13607, new element #2=w13607, new element #3=w13608, new element #4=w13609, new element #5=w13607, new element #6=w13607, new element #7=w13607, new element #8=w13607, new element #9=w13607, new element #10=w13607, new element #11=w13610, new element #12=w13611) -> (w13613:string[][])  [unwired: 1 in]
                        n2492 = call "flot graph for month n year.vi"("BD Date"=w13614, "error in (no error)"=w13616, "Count total"=w13610) -> ("error out"=w13615:errorcluster, "Run-Time Status"=w13612:cluster{"Array 2":timestamp[], dbl[]})  [unwired: 7 in]
                        n2493 = local write "Run-Time Status"(w13612) -> ()
                        n2494 = local write "Table"(w13613) -> ()
                      }
                    }
                  }
                  frame "all" {
                  }
                }
              }
              frame "Maintenance" {
                n2495 = local read "Shift"() -> (w13620:string)
                n2496 = case shown="\"1\"" w13620 {
                  selector: w13620 -> [_ w13993 w14372 w14751 _]
                  tunnel: w13625 -> [w13630 w13998 w14377 w14756 _]
                  tunnel: w13624 -> [w13629 w13997 w14376 w14755 _]
                  tunnel: w13623 -> [w13628 w13996 w14375 w14754 _]
                  tunnel: w13622 -> [w13627 w13995 w14374 w14753 _]
                  tunnel: w13621 -> [w13626 w13994 w14373 w14752 _]
                  frame "ALL", Default {
                    n2497 = flat-sequence {
                      tunnel: w13630 -> [w13742]
                      tunnel: w13629 -> [w13740]
                      tunnel: [w13726] -> w13720
                      tunnel: [w13741] -> w13719
                      tunnel: w13628 -> [_]
                      tunnel: [w13745] -> w13718
                      tunnel: [w13725] -> w13717
                      tunnel: [w13724] -> w13716
                      tunnel: [w13722] -> w13715
                      tunnel: w13627 -> [w13725]
                      tunnel: w13626 -> [w13724]
                      tunnel: ["Where BREAKDOWN_DATE between '%s'and '%s' and BREAKDOWN_STK_HOLD_ID ='%d'  "] -> w13714
                      tunnel: [w13722] -> w13713
                      tunnel: w13720 -> [w13804]
                      tunnel: w13719 -> [w13806]
                      tunnel: w13718 -> [w13802]
                      tunnel: w13717 -> [w13801]
                      tunnel: w13716 -> [w13800]
                      tunnel: [w13803] -> w13712
                      tunnel: [w13805] -> w13711
                      tunnel: [w13802] -> w13710
                      tunnel: [w13792] -> w13709
                      tunnel: [w13798] -> w13708
                      tunnel: [w13801] -> w13707
                      tunnel: [w13800] -> w13706
                      tunnel: w13715 -> [w13797]
                      tunnel: [w13797] -> w13705
                      tunnel: w13714 -> [w13794]
                      tunnel: [w13794] -> w13704
                      tunnel: [w13793] -> w13703
                      tunnel: w13713 -> [w13793]
                      tunnel: w13712 -> [w13832]
                      tunnel: w13711 -> [w13830]
                      tunnel: w13710 -> [w13835]
                      tunnel: w13709 -> [w13834]
                      tunnel: w13708 -> [w13833]
                      tunnel: w13707 -> [w13828]
                      tunnel: w13706 -> [w13827]
                      tunnel: [w13835] -> w13702
                      tunnel: [w13834] -> w13701
                      tunnel: [w13833] -> w13700
                      tunnel: [w13831] -> w13699
                      tunnel: [w13825] -> w13698
                      tunnel: [w13824] -> w13697
                      tunnel: [w13829] -> w13696
                      tunnel: [w13828] -> w13695
                      tunnel: [w13827] -> w13694
                      tunnel: w13705 -> [w13823]
                      tunnel: [w13823] -> w13693
                      tunnel: w13704 -> [w13820]
                      tunnel: [w13820] -> w13692
                      tunnel: [w13819] -> w13691
                      tunnel: w13703 -> [w13819]
                      tunnel: w13702 -> [w13867]
                      tunnel: w13701 -> [w13866]
                      tunnel: w13700 -> [w13865]
                      tunnel: w13699 -> [w13862]
                      tunnel: w13698 -> [w13864]
                      tunnel: w13697 -> [w13863]
                      tunnel: w13696 -> [w13860]
                      tunnel: w13695 -> [w13858]
                      tunnel: w13694 -> [w13857]
                      tunnel: [w13867] -> w13690
                      tunnel: [w13866] -> w13689
                      tunnel: [w13865] -> w13688
                      tunnel: [w13864] -> w13687
                      tunnel: [w13863] -> w13686
                      tunnel: [w13861] -> w13685
                      tunnel: [w13855] -> w13684
                      tunnel: [w13854] -> w13683
                      tunnel: [w13859] -> w13682
                      tunnel: [w13858] -> w13681
                      tunnel: [w13857] -> w13680
                      tunnel: w13693 -> [w13853]
                      tunnel: [w13853] -> w13679
                      tunnel: w13692 -> [w13850]
                      tunnel: [w13850] -> w13678
                      tunnel: [w13849] -> w13677
                      tunnel: w13691 -> [w13849]
                      tunnel: w13690 -> [w13888]
                      tunnel: w13689 -> [w13887]
                      tunnel: w13688 -> [w13886]
                      tunnel: w13687 -> [w13885]
                      tunnel: w13686 -> [w13884]
                      tunnel: w13685 -> [w13881]
                      tunnel: w13684 -> [w13883]
                      tunnel: w13683 -> [w13882]
                      tunnel: w13682 -> [w13880]
                      tunnel: w13681 -> [w13877]
                      tunnel: w13680 -> [w13876]
                      tunnel: [w13888] -> w13676
                      tunnel: [w13887] -> w13675
                      tunnel: [w13886] -> w13674
                      tunnel: [w13885] -> w13673
                      tunnel: [w13884] -> w13672
                      tunnel: [w13883] -> w13671
                      tunnel: [w13882] -> w13670
                      tunnel: [w13879] -> w13669
                      tunnel: [w13878] -> w13668
                      tunnel: [w13874] -> w13667
                      tunnel: [w13873] -> w13666
                      tunnel: [w13877] -> w13665
                      tunnel: [w13876] -> w13664
                      tunnel: w13679 -> [w13872]
                      tunnel: [w13872] -> w13663
                      tunnel: w13678 -> [w13869]
                      tunnel: [w13869] -> w13662
                      tunnel: [w13868] -> w13661
                      tunnel: w13677 -> [w13868]
                      tunnel: w13676 -> [w13923]
                      tunnel: w13675 -> [w13922]
                      tunnel: w13674 -> [w13921]
                      tunnel: w13673 -> [w13920]
                      tunnel: w13672 -> [w13919]
                      tunnel: w13671 -> [w13918]
                      tunnel: w13670 -> [w13917]
                      tunnel: w13669 -> [w13912]
                      tunnel: w13668 -> [w13914]
                      tunnel: w13667 -> [w13916]
                      tunnel: w13666 -> [w13915]
                      tunnel: w13665 -> [w13909]
                      tunnel: w13664 -> [w13910]
                      tunnel: [w13923] -> w13660
                      tunnel: [w13922] -> w13659
                      tunnel: [w13921] -> w13658
                      tunnel: [w13920] -> w13657
                      tunnel: [w13919] -> w13656
                      tunnel: [w13918] -> w13655
                      tunnel: [w13917] -> w13654
                      tunnel: [w13916] -> w13653
                      tunnel: [w13915] -> w13652
                      tunnel: [w13913] -> w13651
                      tunnel: [w13911] -> w13650
                      tunnel: [w13907] -> w13649
